vi "TDC_DAQV28_Paralled_muon.vi"(7 "address":string[](array[string])=["192.168.10.20"], 8 "error in (no error)":errorcluster, 9 "stop":bool, 10 "save data":bool=TRUE, 11 "SMA mode":bool) -> (0 "error out 3":errorcluster, 2 "csv path":path=path "G:/tdc/2017/data/test_20250303_062615.csv", 3 "rate":dbl=1.0935487223592613)   [LabVIEW 2017]
uses:
  gloabal.vi
  <vilib>/Utility/file.llb/Write Delimited Spreadsheet (DBL).vi
  <vilib>/Utility/file.llb/Write Delimited Spreadsheet (I64).vi
panel:
  out "cal 3":u32[](graph)=[0, 0, 0, 0, 0, 0, 0, 0, 0, 0, 0, 0, 0, 0, 0, 0, 0, 0, 0, 0, 0, 0, 0, 0, 0, 0, 0, 0, 0, 0, 0, 0, 0, 0, 0, 0, 0, 0, 0, 0, 0, 0, 0, 0, 0, 0, 0, 0, 0, 0, 0, 0, 0, 0, 0, 0, 0, 0, 0, 0, 0, 0, 0, 0, 0, 0, 0, 0, 0, 0, 0, 0, 0, 0, 0, 0, 0, 0, 0, 0, 0, 0, 0, 0, 0, 0, 0, 0, 0, 0, 0, 0, 0, 0, 0, 0, 0, 0, 0, 0, 0, 0, 0, 0, 0, 0, 0, 0, 0, 0, 0, 0, 0, 0, 0, 0, 0, 0, 0, 0, 0, 0, 0, 0, 0, 0, 0, 0, 0, 0, 0, 0, 0, 0, 0, 0, 0, 0, 0, 0, 0, 0, 0, 0, 0, 0, 0, 0, 0, 0, 0, 0, 0, 0, 0, 0, 0, 0, 0, 0, 0, 0, 0, 0, 0, 15, 3, 1, 14, 3, 31, 20, 16, 6, 1, 18, 12, 4, 29, 10, 8, 29, 2, 14, 4, 25, 7, 24, 4, 0, 1, 5, 8, 18, 22, 0, 4, 5, 0, 12, 9, 9, 20, 21, 4, 10, 13, 5, 21, 13, 14, 2, 6, 13, 1, 3, 5, 10, 20, 2, 3, 4, 3, 4, 2, 20, 13, 2, 5, 1, 3, 12, 4, 1, 14, 7, 5, 4, 1, 10, 2, 21, 14, 2, 5, 10, 4, 0, 11, 19, 6, 4, 1, 37, 1, 4, 2, 1, 10, 13, 4, 8, 10, 6, 9, 2, 0, 6, 8, 12, 3, 21, 5, 7, 8, 2, 3, 7, 17, 6, 5, 6, 4, 6, 0, 2, 1, 3, 10, 33, 7, 2, 6, 3, 7, 3, 2, 0, 12, 10, 11, 13, 13, 7, 3, 9, 6, 16, 0, 13, 5, 6, 3, 0, 5, 5, 7, 1, 10, 7, 13, 14, 5, 1, 12, 7, 1, 10, 2, 1, 14, 18, 13, 11, 4, 6, 9, 22, 11, 9, 2, 2, 8, 14, 4, 4, 6, 12, 13, 3, 9, 5, 5, 1, 5, 11, 18, 3, 0, 5, 4, 6, 7, 6, 1, 13, 5, 1, 2, 2, 1, 4, 12, 7, 3, 2, 3, 9, 11, 1, 20, 3, 4, 5, 5, 3, 5, 8, 5, 3, 26, 14, 6, 1, 3, 12, 12, 4, 23, 10, 3, 4, 4, 10, 3, 5, 4, 2, 14, 5, 15, 20, 1, 5, 1, 20, 6, 1, 3, 13, 21, 12, 7, 4, 1, 5, 30, 11, 2, 4, 0, 12, 7, 10, 3, 2, 25, 6, 1, 3, 6, 3, 8, 37, 4, 6, 2, 2, 4, 3, 5, 6, 13, 6, 9, 22, 1, 3, 7, 7, 4, 8, 33, 2, 1, 15, 3, 8, 23, 21, 2, 2, 27, 13, 3, 5, 10, 4, 18, 5, 5, 8, 0, 1, 8, 12, 4, 3, 0, 4, 8, 4, 7, 4, 2, 11, 13, 3, 0, 7, 5, 3, 4, 8, 4, 20, 2, 13, 4, 8, 6, 17, 4, 2, 1, 15, 2, 15, 5, 19, 0, 4, 15, 4, 16, 11, 1, 16, 4, 6, 6, 5, 7, 3, 9, 15, 3, 6, 3, 13, 5, 7, 3, 27, 2, 0, 21, 1, 4, 1, 4, 5, 3, 10, 7, 3, 6, 4, 18, 21, 7, 6, 7, 7, 12, 6, 9, 8, 11, 12, 13, 2, 2, 5, 4, 7, 52, 3, 5, 8, 7, 10, 4, 4, 6, 5, 18, 0, 3, 6, 1, 9, 5, 19, 13, 24, 12, 4, 4, 15, 6, 41, 3, 8, 5, 17, 26, 8, 7, 20, 2, 5, 12, 10, 10, 12, 9, 17, 6, 3, 1, 5, 3, 7, 8, 4, 10, 5, 10, 7, 1, 2, 14, 7, 25, 3, 0, 0, 0, 5, 21, 8, 14, 4, 10, 2, 3, 2, 4, 8, 12, 3, 6, 8, 3, 4, 3, 20, 5, 6, 7, 8, 11, 2, 8, 6, 5, 15, 17, 10, 10, 3, 3, 9, 18, 7, 7, 3, 5, 5, 5, 2, 2, 2, 4, 1, 0, 42, 3, 14, 4, 3, 5, 2, 7, 4, 2, 7, 5, 22, 4, 3, 17, 3, 5, 8, 19, 7, 5, 0, 3, 4, 10, 1, 8, 2, 2, 13, 23, 4, 9, 5, 0, 0, 0, 27, 2, 16, 11, 15, 3, 0, 18, 2, 8, 29, 19, 6, 7, 2, 6, 12, 1, 13, 2, 7, 5, 11, 8, 5, 6, 6, 19, 2, 4, 0, 7, 22, 13, 3, 7, 3, 8, 11, 0, 3, 26, 6, 5, 5, 6, 4, 10, 17, 16, 4, 3, 4, 3, 4, 21, 8, 10, 10, 7, 0, 9, 9, 2, 10, 10, 2, 9, 9, 4, 14, 5, 5, 4, 18, 6, 3, 0, 4, 1, 20, 2, 33, 4, 1, 2, 1, 20, 6, 3, 11, 10, 2, 1, 13, 9, 6, 1, 0, 0, 0, 0, 0, 0, 0, 0, 0, 0, 0, 0, 0, 0, 0, 0, 0, 0, 0, 0, 0, 0, 0, 0, 0, 0, 0, 0, 0, 0, 0, 0, 0, 0, 0, 0, 0, 0, 0, 0, 0, 0, 0, 0, 0, 0, 0, 0, 0, 0, 0, 0, 0, 0, 0, 0, 0, 0, 0, 0, 0, 0, 0, 0, 0, 0, 0, 0, 0, 0, 0, 0, 0, 0, 0, 0, 0, 0, 0, 0, 0, 0, 0, 0, 0, 0, 0, 0, 0, 0, 0, 0, 0, 0, 0, 0, 0, 0, 0, 0, 0, 0, 0, 0, 0, 0, 0, 0, 0, 0, 0, 0, 0, 0, 0, 0, 0, 0, 0, 0, 0, 0, 0, 0, 0, 0, 0, 0, 0, 0, 0, 0, 0, 0, 0, 0, 0, 0, 0, 0, 0, 0, 0, 0, 0, 0, 0, 0, 0, 0, 0, 0, 0, 0, 0, 0, 0, 0, 0, 0, 0, 0, 0, 0, 0, 0, 0, 0, 0, 0, 0, 0, 0, 0, 0, 0, 0, 0, 0, 0, 0, 0, 0, 0, 0, 0, 0, 0, 0, 0, 0, 0, 0, 0, 0, 0, 0, 0, 0, 0, 0, 0, 0, 0, 0, 0, 0, 0, 0, 0, 0, 0, 0, 0, 0, 0, 0, 0, 0, 0, 0, 0, 0, 0, 0, 0, 0, 0, 0, 0, 0, 0, 0, 0, 0, 0, 0, 0, 0, 0, 0, 0, 0, 0, 0, 0, 0, 0, 0, 0, 0, 0, 0, 0, 0, 0, 0, 0, 0, 0, 0, 0, 0, 0, 0, 0, 0, 0, 0, 0, 0, 0, 0, 0, 0, 0, 0, 0, 0, 0, 0, 0, 0, 0, 0, 0, 0, 0, 0, 0, 0, 0, 0, 0, 0, 0, 0, 0, 0, 0, 0, 0, 0, 0, 0, 0, 0, 0, 0, 0, 0, 0, 0, 0, 0, 0, 0, 0, 0, 0, 0, 0, 0, 0, 0, 0, 0, 0, 0, 0, 0, 0, 0, 0, 0, 0, 0, 0, 0, 0, 0, 0, 0, 0, 0, 0, 0, 0, 0, 0, 0, 0, 0, 0, 0, 0, 0, 0, 0, 0, 0, 0, 0, 0, 0, 0, 0, 0, 0, 0, 0, 0, 0, 0, 0, 0, 0, 0, 0, 0, 0, 0, 0, 0, 0, 0, 0, 0, 0, 0, 0, 0, 0, 0, 0, 0, 0, 0, 0, 0, 0, 0, 0, 0, 0, 0, 0, 0, 0, 0, 0, 0, 0, 0, 0, 0, 0, 0, 0, 0, 0, 0, 0, 0, 0, 0, 0, 0, 0, 0, 0, 0, 0, 0, 0, 0, 0, 0, 0, 0, 0, 0, 0, 0, 0, 0, 0, 0, 0, 0, 0, 0, 0, 0, 0, 0, 0, 0, 0, 0, 0, 0, 0, 0, 0, 0, 0, 0, 0, 0, 0, 0, 0, 0, 0, 0, 0, 0, 0, 0, 0, 0, 0, 0, 0, 0, 0, 0, 0, 0, 0, 0, 0, 0, 0, 0, 0, 0, 0, 0, 0, 0, 0, 0, 0, 0, 0, 0, 0, 0, 0, 0, 0, 0, 0, 0, 0, 0, 0, 0, 0, 0, 0, 0, 0, 0, 0, 0, 0, 0, 0, 0, 0, 0, 0, 0, 0, 0, 0, 0, 0, 0, 0, 0, 0, 0, 0, 0, 0, 0, 0, 0, 0, 0, 0, 0, 0, 0, 0, 0, 0, 0, 0, 0, 0, 0, 0, 0, 0, 0, 0, 0, 0, 0, 0, 0, 0, 0, 0, 0, 0, 0, 0, 0, 0, 0, 0, 0, 0, 0, 0, 0, 0, 0, 0, 0, 0, 0, 0, 0, 0, 0, 0, 0, 0, 0, 0, 0, 0, 0, 0, 0, 0, 0, 0, 0, 0, 0, 0, 0, 0, 0, 0, 0, 0, 0, 0, 0, 0, 0, 0, 0, 0, 0, 0, 0, 0, 0, 0, 0, 0, 0, 0, 0, 0, 0, 0, 0, 0, 0, 0, 0, 0, 0, 0, 0, 0, 0, 0, 0, 0, 0, 0, 0, 0, 0, 0, 0, 0, 0, 0, 0, 0, 0, 0, 0, 0, 0, 0, 0, 0, 0, 0, 0, 0, 0, 0, 0, 0, 0, 0, 0, 0, 0, 0, 0, 0, 0, 0, 0, 0, 0, 0, 0, 0, 0, 0, 0, 0, 0, 0, 0, 0, 0, 0, 0, 0, 0, 0, 0, 0, 0, 0, 0, 0, 0, 0, 0, 0, 0, 0, 0, 0, 0, 0, 0, 0, 0, 0, 0, 0, 0, 0, 0, 0, 0, 0, 0, 0, 0, 0, 0, 0, 0, 0, 0, 0, 0, 0, 0, 0, 0, 0, 0, 0, 0, 0, 0, 0, 0, 0, 0, 0, 0, 0, 0, 0, 0, 0, 0, 0, 0, 0, 0, 0, 0, 0, 0, 0, 0, 0, 0, 0, 0, 0, 0, 0, 0, 0, 0, 0, 0, 0, 0, 0, 0, 0, 0, 0, 0, 0, 0, 0, 0, 0, 0, 0, 0, 0, 0, 0, 0, 0, 0, 0, 0, 0, 0, 0, 0, 0, 0, 0, 0, 0, 0, 0, 0, 0, 0, 0, 0, 0, 0, 0, 0, 0, 0, 0, 0, 0, 0, 0, 0, 0, 0, 0, 0, 0, 0, 0, 0, 0, 0, 0, 0, 0, 0, 0, 0, 0, 0, 0, 0, 0, 0, 0, 0, 0, 0, 0, 0, 0, 0, 0, 0, 0, 0, 0, 0, 0, 0, 0, 0, 0, 0, 0, 0, 0, 0, 0, 0, 0, 0, 0, 0, 0, 0, 0, 0, 0, 0, 0, 0, 0, 0, 0, 0, 0, 0, 0, 0, 0, 0, 0, 0, 0, 0, 0, 0, 0, 0, 0, 0, 0, 0, 0, 0, 0, 0, 0, 0, 0, 0, 0, 0, 0, 0, 0, 0, 0, 0, 0, 0, 0, 0, 0, 0, 0, 0, 0, 0, 0, 0, 0, 0, 0, 0, 0, 0, 0, 0, 0, 0, 0, 0, 0, 0, 0, 0, 0, 0, 0, 0, 0, 0, 0, 0, 0, 0, 0, 0, 0, 0, 0, 0, 0, 0, 0, 0, 0, 0, 0, 0, 0, 0, 0, 0, 0, 0, 0, 0, 0, 0, 0, 0, 0, 0, 0, 0, 0, 0, 0, 0, 0, 0, 0, 0, 0, 0, 0, 0, 0, 0, 0, 0, 0, 0, 0, 0, 0, 0, 0, 0, 0, 0, 0, 0, 0, 0, 0, 0, 0, 0, 0, 0, 0, 0, 0, 0, 0, 0, 0, 0, 0, 0, 0, 0, 0, 0, 0, 0, 0, 0, 0, 0, 0, 0, 0, 0, 0, 0, 0, 0, 0, 0, 0, 0, 0, 0, 0, 0, 0, 0, 0, 0, 0, 0, 0, 0, 0, 0, 0, 0, 0, 0, 0, 0, 0, 0, 0, 0, 0, 0, 0, 0, 0, 0, 0, 0, 0, 0, 0, 0, 0, 0, 0, 0, 0, 0, 0, 0, 0, 0, 0, 0, 0, 0, 0, 0, 0, 0, 0, 0, 0, 0, 0, 0, 0, 0, 0, 0, 0, 0, 0, 0, 0, 0, 0, 0, 0, 0, 0, 0, 0, 0, 0, 0, 0, 0, 0, 0, 0, 0, 0, 0, 0, 0, 0, 0, 0, 0, 0, 0, 0, 0, 0, 0, 0, 0, 0, 0, 0, 0, 0, 0, 0, 0, 0, 0, 0, 0, 0, 0, 0, 0, 0, 0, 0, 0, 0, 0, 0, 0, 0, 0, 0, 0, 0, 0, 0, 0, 0, 0, 0]
  out "x+y":u64
  out "channel number 3":u64 format="%x"
  in  "coarse counter width":u16(ring) items=["29", "48"]
  out "name (unnamed)":string
  out "error out 5":errorcluster
  in  "timeout":dbl=300.0
  out "DAC":dbl=8094.0
  out "Out":u8=3 format="%.0x"
  out "fine 4":u64=356036515840 format="%x"
  out "fine 3":u64=1390767640 format="%x"
  out "channel number 2":u64 format="%x"
  out "substring 3":string
  out "fine 2":u64=347691910 format="%x"
  out "substring 2":string
  out "substring":string
  in  "gps":bool
  out "Year":string="2025"
  in  "factor":i32=128
  in  "displayCR":bool=TRUE
  in  "Counter Setting":dbl=100000.0 format="%#_13g"
  in  "replace dat":bool
  in  "append csv":bool=TRUE
  out "element":string
  out "fine":u64=749 format="%x"
  in  "UDP Config":bool=TRUE
  in  "data  path":path=path "G:/tdc/2017/data"
  out "cal 2":u64[](graph)
  in  "Thresholds (mV)":dbl[](array[numeric])=[580.0, 580.0, 580.0, 580.0, 600.0, 600.0, 600.0, 600.0, 580.0, 580.0, 600.0, 600.0, 600.0, 600.0, 600.0, 600.0, 580.0, 580.0, 600.0, 600.0, 600.0, 600.0, 600.0, 600.0, 580.0, 580.0, 600.0, 600.0, 600.0, 600.0, 600.0, 600.0, 600.0, 600.0, 600.0, 600.0, 600.0, 600.0, 600.0, 600.0, 600.0, 600.0, 600.0, 600.0, 600.0, 600.0, 600.0, 600.0, 600.0, 600.0, 600.0, 600.0, 600.0, 600.0, 600.0, 600.0, 600.0, 600.0, 600.0, 600.0, 600.0, 600.0, 600.0, 600.0]
  out "error out 2":errorcluster
  in  "display":bool=TRUE
  in  "Thresholds":dbl=-0.03
  in  "one key for threshold":bool=TRUE
  in  "RST":bool
  in  "通道数量":i32=128
  out "Cal Table":u32[](array[numeric])=[100002, 100002, 0, 0, 0, 0, 0, 0, 0, 0, 0, 0, 0, 0, 0, 0, 0, 0, 0, 0, 0, 0, 0, 0, 0, 0, 0, 0, 0, 0, 0, 0, 0, 0, 0, 0, 0, 0, 0, 0, 0, 0, 0, 0, 0, 0, 0, 0, 0, 0, 0, 0, 0, 0, 0, 0, 0, 0, 0, 0, 0, 0, 0, 0, 0, 0, 0, 0, 0, 0, 0, 0, 0, 0, 0, 0, 0, 0, 0, 0, 0, 0, 0, 0, 0, 0, 0, 0, 0, 0, 0, 0, 0, 0, 0, 0, 0, 0, 100002, 100002, 0, 0, 0, 0, 0, 0, 0, 0, 0, 0, 0, 0, 0, 0, 0, 0, 0, 0, 0, 0, 0, 0, 0, 0, 0, 0, 0, 0]
  in  "channel for cal":i32
  out "channel number":u64
  out "Calibration Counter":i32=100000
  out "Event index":i32=97959
  out "cal":u32[](graph)=[0, 0, 0, 0, 0, 0, 0, 0, 0, 0, 0, 0, 0, 0, 0, 0, 0, 0, 0, 0, 0, 0, 0, 0, 0, 0, 0, 0, 0, 0, 0, 0, 0, 0, 0, 0, 0, 0, 0, 0, 0, 0, 0, 0, 0, 0, 0, 0, 0, 0, 0, 0, 0, 0, 0, 0, 0, 0, 0, 0, 0, 0, 0, 0, 0, 0, 0, 0, 0, 0, 0, 0, 0, 0, 0, 0, 0, 0, 0, 0, 0, 0, 0, 0, 0, 0, 0, 0, 0, 0, 0, 0, 0, 0, 0, 0, 0, 0, 0, 0, 0, 0, 0, 0, 0, 0, 0, 0, 0, 0, 0, 0, 0, 0, 0, 0, 0, 0, 0, 0, 0, 0, 0, 0, 0, 0, 0, 0, 0, 0, 0, 0, 0, 0, 0, 0, 0, 0, 0, 0, 0, 0, 0, 0, 0, 0, 0, 0, 0, 0, 0, 0, 0, 0, 0, 0, 0, 0, 0, 0, 0, 0, 0, 0, 0, 15, 511, 47, 47, 496, 61, 99, 729, 29, 42, 171, 747, 96, 51, 42, 172, 695, 176, 314, 56, 529, 577, 49, 39, 32, 59, 217, 100, 54, 274, 367, 65, 147, 131, 182, 81, 199, 147, 352, 77, 542, 71, 254, 473, 91, 290, 270, 470, 39, 34, 220, 292, 32, 36, 306, 91, 30, 60, 270, 84, 115, 92, 342, 59, 193, 51, 55, 166, 178, 68, 201, 77, 48, 251, 157, 58, 175, 144, 73, 238, 174, 189, 202, 77, 49, 49, 85, 297, 134, 135, 191, 31, 343, 221, 39, 85, 162, 328, 62, 89, 210, 178, 65, 221, 260, 157, 46, 41, 35, 131, 307, 87, 392, 108, 46, 60, 293, 50, 28, 167, 101, 165, 43, 61, 148, 522, 39, 60, 263, 49, 52, 418, 91, 68, 40, 20, 504, 53, 95, 56, 124, 80, 60, 291, 176, 200, 307, 95, 332, 51, 42, 79, 81, 128, 130, 107, 114, 54, 243, 271, 151, 90, 157, 326, 162, 89, 139, 327, 44, 132, 379, 66, 138, 71, 729, 73, 135, 130, 269, 267, 206, 92, 141, 79, 58, 103, 46, 162, 368, 174, 84, 171, 248, 161, 88, 87, 85, 141, 71, 79, 100, 248, 53, 62, 46, 50, 29, 51, 151, 324, 134, 72, 55, 273, 116, 57, 432, 69, 101, 121, 112, 68, 129, 194, 50, 95, 235, 79, 432, 83, 320, 56, 85, 118, 185, 276, 83, 46, 247, 134, 161, 99, 82, 54, 346, 250, 66, 379, 111, 58, 47, 307, 58, 79, 133, 244, 54, 262, 133, 46, 43, 39, 274, 241, 171, 55, 222, 121, 72, 279, 53, 50, 69, 528, 61, 153, 48, 220, 139, 41, 384, 59, 142, 79, 150, 65, 43, 287, 51, 216, 69, 111, 314, 50, 328, 87, 107, 247, 222, 49, 113, 194, 307, 485, 52, 60, 292, 98, 760, 36, 82, 65, 80, 90, 182, 181, 48, 192, 40, 156, 51, 325, 87, 36, 31, 44, 140, 97, 82, 144, 162, 67, 335, 57, 34, 44, 107, 46, 49, 157, 326, 231, 52, 48, 325, 105, 61, 219, 47, 357, 66, 68, 245, 77, 106, 285, 61, 245, 39, 43, 236, 326, 164, 131, 73, 165, 77, 225, 56, 62, 45, 422, 137, 93, 81, 169, 47, 198, 173, 350, 60, 357, 57, 32, 55, 64, 54, 64, 147, 199, 199, 92, 169, 312, 172, 158, 231, 65, 129, 68, 243, 77, 214, 57, 316, 70, 86, 59, 128, 51, 39, 930, 119, 134, 78, 46, 106, 248, 87, 93, 90, 320, 90, 60, 76, 239, 138, 140, 375, 323, 460, 154, 50, 67, 245, 237, 687, 62, 74, 111, 420, 292, 99, 335, 396, 57, 225, 111, 125, 191, 131, 151, 340, 112, 74, 88, 108, 142, 215, 212, 62, 224, 110, 55, 62, 110, 67, 75, 331, 263, 111, 107, 156, 80, 35, 160, 178, 377, 128, 77, 200, 62, 55, 60, 185, 235, 153, 63, 102, 299, 52, 72, 427, 135, 66, 95, 93, 146, 410, 54, 135, 78, 207, 103, 114, 94, 379, 159, 137, 422, 82, 64, 49, 43, 48, 73, 426, 60, 46, 37, 39, 50, 329, 413, 120, 95, 108, 29, 66, 59, 254, 54, 62, 160, 117, 230, 100, 119, 290, 131, 164, 113, 145, 149, 109, 172, 90, 127, 129, 161, 60, 153, 140, 107, 110, 117, 131, 297, 70, 47, 399, 156, 187, 68, 61, 212, 125, 427, 52, 289, 198, 138, 147, 346, 170, 168, 330, 74, 71, 89, 314, 331, 132, 133, 97, 154, 80, 111, 135, 270, 207, 206, 349, 111, 57, 278, 56, 155, 199, 230, 49, 176, 311, 128, 140, 146, 205, 111, 202, 158, 309, 108, 180, 95, 107, 237, 174, 119, 149, 86, 87, 234, 78, 88, 101, 101, 247, 99, 131, 235, 140, 122, 39, 83, 64, 241, 51, 34, 52, 104, 13, 43, 35, 30, 7, 0, 0, 1, 0, 0, 0, 0, 0, 0, 0, 0, 0, 0, 0, 0, 0, 0, 0, 0, 0, 0, 0, 0, 0, 0, 0, 0, 0, 0, 0, 0, 0, 0, 0, 0, 0, 0, 0, 0, 0, 0, 0, 0, 0, 0, 0, 0, 0, 0, 0, 0, 0, 0, 0, 0, 0, 0, 0, 0, 0, 0, 0, 0, 0, 0, 0, 0, 0, 0, 0, 0, 0, 0, 0, 0, 0, 0, 0, 0, 0, 0, 0, 0, 0, 0, 0, 0, 0, 0, 0, 0, 0, 0, 0, 0, 0, 0, 0, 0, 0, 0, 0, 0, 0, 0, 0, 0, 0, 0, 0, 0, 0, 0, 0, 0, 0, 0, 0, 0, 0, 0, 0, 0, 0, 0, 0, 0, 0, 0, 0, 0, 0, 0, 0, 0, 0, 0, 0, 0, 0, 0, 0, 0, 0, 0, 0, 0, 0, 0, 0, 0, 0, 0, 0, 0, 0, 0, 0, 0, 0, 0, 0, 0, 0, 0, 0, 0, 0, 0, 0, 0, 0, 0, 0, 0, 0, 0, 0, 0, 0, 0, 0, 0, 0, 0, 0, 0, 0, 0, 0, 0, 0, 0, 0, 0, 0, 0, 0, 0, 0, 0, 0, 0, 0, 0, 0, 0, 0, 0, 0, 0, 0, 0, 0, 0, 0, 0, 0, 0, 0, 0, 0, 0, 0, 0, 0, 0, 0, 0, 0, 0, 0, 0, 0, 0, 0, 0, 0, 0, 0, 0, 0, 0, 0, 0, 0, 0, 0, 0, 0, 0, 0, 0, 0, 0, 0, 0, 0, 0, 0, 0, 0, 0, 0, 0, 0, 0, 0, 0, 0, 0, 0, 0, 0, 0, 0, 0, 0, 0, 0, 0, 0, 0, 0, 0, 0, 0, 0, 0, 0, 0, 0, 0, 0, 0, 0, 0, 0, 0, 0, 0, 0, 0, 0, 0, 0, 0, 0, 0, 0, 0, 0, 0, 0, 0, 0, 0, 0, 0, 0, 0, 0, 0, 0, 0, 0, 0, 0, 0, 0, 0, 0, 0, 0, 0, 0, 0, 0, 0, 0, 0, 0, 0, 0, 0, 0, 0, 0, 0, 0, 0, 0, 0, 0, 0, 0, 0, 0, 0, 0, 0, 0, 0, 0, 0, 0, 0, 0, 0, 0, 0, 0, 0, 0, 0, 0, 0, 0, 0, 0, 0, 0, 0, 0, 0, 0, 0, 0, 0, 0, 0, 0, 0, 0, 0, 0, 0, 0, 0, 0, 0, 0, 0, 0, 0, 0, 0, 0, 0, 0, 0, 0, 0, 0, 0, 0, 0, 0, 0, 0, 0, 0, 0, 0, 0, 0, 0, 0, 0, 0, 0, 0, 0, 0, 0, 0, 0, 0, 0, 0, 0, 0, 0, 0, 0, 0, 0, 0, 0, 0, 0, 0, 0, 0, 0, 0, 0, 0, 0, 0, 0, 0, 0, 0, 0, 0, 0, 0, 0, 0, 0, 0, 0, 0, 0, 0, 0, 0, 0, 0, 0, 0, 0, 0, 0, 0, 0, 0, 0, 0, 0, 0, 0, 0, 0, 0, 0, 0, 0, 0, 0, 0, 0, 0, 0, 0, 0, 0, 0, 0, 0, 0, 0, 0, 0, 0, 0, 0, 0, 0, 0, 0, 0, 0, 0, 0, 0, 0, 0, 0, 0, 0, 0, 0, 0, 0, 0, 0, 0, 0, 0, 0, 0, 0, 0, 0, 0, 0, 0, 0, 0, 0, 0, 0, 0, 0, 0, 0, 0, 0, 0, 0, 0, 0, 0, 0, 0, 0, 0, 0, 0, 0, 0, 0, 0, 0, 0, 0, 0, 0, 0, 0, 0, 0, 0, 0, 0, 0, 0, 0, 0, 0, 0, 0, 0, 0, 0, 0, 0, 0, 0, 0, 0, 0, 0, 0, 0, 0, 0, 0, 0, 0, 0, 0, 0, 0, 0, 0, 0, 0, 0, 0, 0, 0, 0, 0, 0, 0, 0, 0, 0, 0, 0, 0, 0, 0, 0, 0, 0, 0, 0, 0, 0, 0, 0, 0, 0, 0, 0, 0, 0, 0, 0, 0, 0, 0, 0, 0, 0, 0, 0, 0, 0, 0, 0, 0, 0, 0, 0, 0, 0, 0, 0, 0, 0, 0, 0, 0, 0, 0, 0, 0, 0, 0, 0, 0, 0, 0, 0, 0, 0, 0, 0, 0, 0, 0, 0, 0, 0, 0, 0, 0, 0, 0, 0, 0, 0, 0, 0, 0, 0, 0, 0, 0, 0, 0, 0, 0, 0, 0, 0, 0, 0, 0, 0, 0, 0, 0, 0, 0, 0, 0, 0, 0, 0, 0, 0, 0, 0, 0, 0, 0, 0, 0, 0, 0, 0, 0, 0, 0, 0, 0, 0, 0, 0, 0, 0, 0, 0, 0, 0, 0, 0, 0, 0, 0, 0, 0, 0, 0, 0, 0, 0, 0, 0, 0, 0, 0, 0, 0, 0, 0, 0, 0, 0, 0, 0, 0, 0, 0, 0, 0, 0, 0, 0, 0, 0, 0, 0, 0, 0, 0, 0, 0, 0, 0, 0, 0, 0, 0, 0, 0, 0, 0, 0, 0, 0, 0, 0, 0, 0, 0, 0, 0, 0, 0, 0, 0, 0, 0, 0, 0, 0, 0, 0, 0, 0, 0, 0, 0, 0, 0, 0, 0, 0, 0, 0, 0, 0, 0, 0, 0, 0, 0, 0, 0, 0, 0, 0, 0, 0, 0, 0, 0, 0, 0, 0, 0, 0, 0, 0, 0, 0, 0, 0, 0, 0, 0, 0, 0, 0, 0, 0, 0, 0, 0, 0, 0, 0, 0, 0, 0, 0, 0, 0, 0, 0, 0, 0, 0, 0, 0, 0, 0, 0, 0, 0, 0, 0, 0, 0, 0, 0, 0, 0, 0, 0, 0, 0, 0, 0, 0, 0, 0, 0, 0, 0, 0, 0, 0, 0, 0, 0, 0, 0, 0, 0, 0, 0, 0, 0, 0, 0, 0, 0, 0, 0, 0, 0, 0, 0, 0, 0, 0, 0, 0, 0, 0, 0, 0, 0, 0, 0, 0, 0, 0, 0, 0, 0, 0, 0, 0, 0, 0, 0, 0, 0, 0, 0, 0, 0, 0, 0, 0, 0, 0, 0, 0, 0, 0, 0, 0, 0, 0, 0, 0, 0, 0, 0, 0, 0, 0, 0, 0, 0, 0, 0, 0, 0, 0, 0, 0, 0, 0, 0, 0, 0, 0, 0, 0, 0, 0, 0, 0, 0, 0, 0, 0, 0, 0, 0, 0, 0, 0, 0, 0, 0, 0, 0, 0, 0, 0, 0, 0, 0, 0, 0, 0, 0, 0, 0, 0, 0, 0, 0, 0, 0, 0, 0, 0, 0, 0, 0, 0, 0, 0, 0, 0, 0, 0, 0, 0, 0, 0, 0, 0, 0, 0, 0, 0, 0, 0, 0, 0, 0, 0, 0, 0, 0, 0, 0, 0, 0, 0, 0, 0, 0, 0, 0, 0, 0, 0, 0, 0, 0, 0, 0, 0, 0, 0, 0, 0, 0, 0, 0, 0, 0, 0, 0, 0, 0, 0, 0, 0, 0, 0, 0, 0, 0, 0, 0, 0, 0, 0, 0, 0, 0, 0, 0, 0, 0, 0, 0, 0, 0, 0, 0, 0, 0, 0, 0, 0, 0, 0, 0, 0, 0, 0, 0, 0, 0, 0, 0, 0, 0, 0, 0, 0, 0, 0, 0, 0, 0, 0, 0, 0, 0, 0, 0, 0, 0, 0, 0, 0, 0, 0, 0, 0, 0, 0, 0, 0, 0, 0, 0, 0, 0, 0, 0, 0, 0, 0, 0, 0, 0, 0, 0, 0, 0, 0, 0, 0, 0, 0, 0, 0, 0, 0, 0, 0, 0, 0, 0, 0, 0, 0, 0, 0, 0, 0, 0, 0, 0, 0, 0, 0, 0, 0]
  out "error out":errorcluster
  out "appended path":path=path "G:/tdc/2017/data/test_20250303_062615.dat"
  in  "filename":string="test"
  in  "Events":i32=110000 min=1
  in  "timeout (ms)":i32=10000
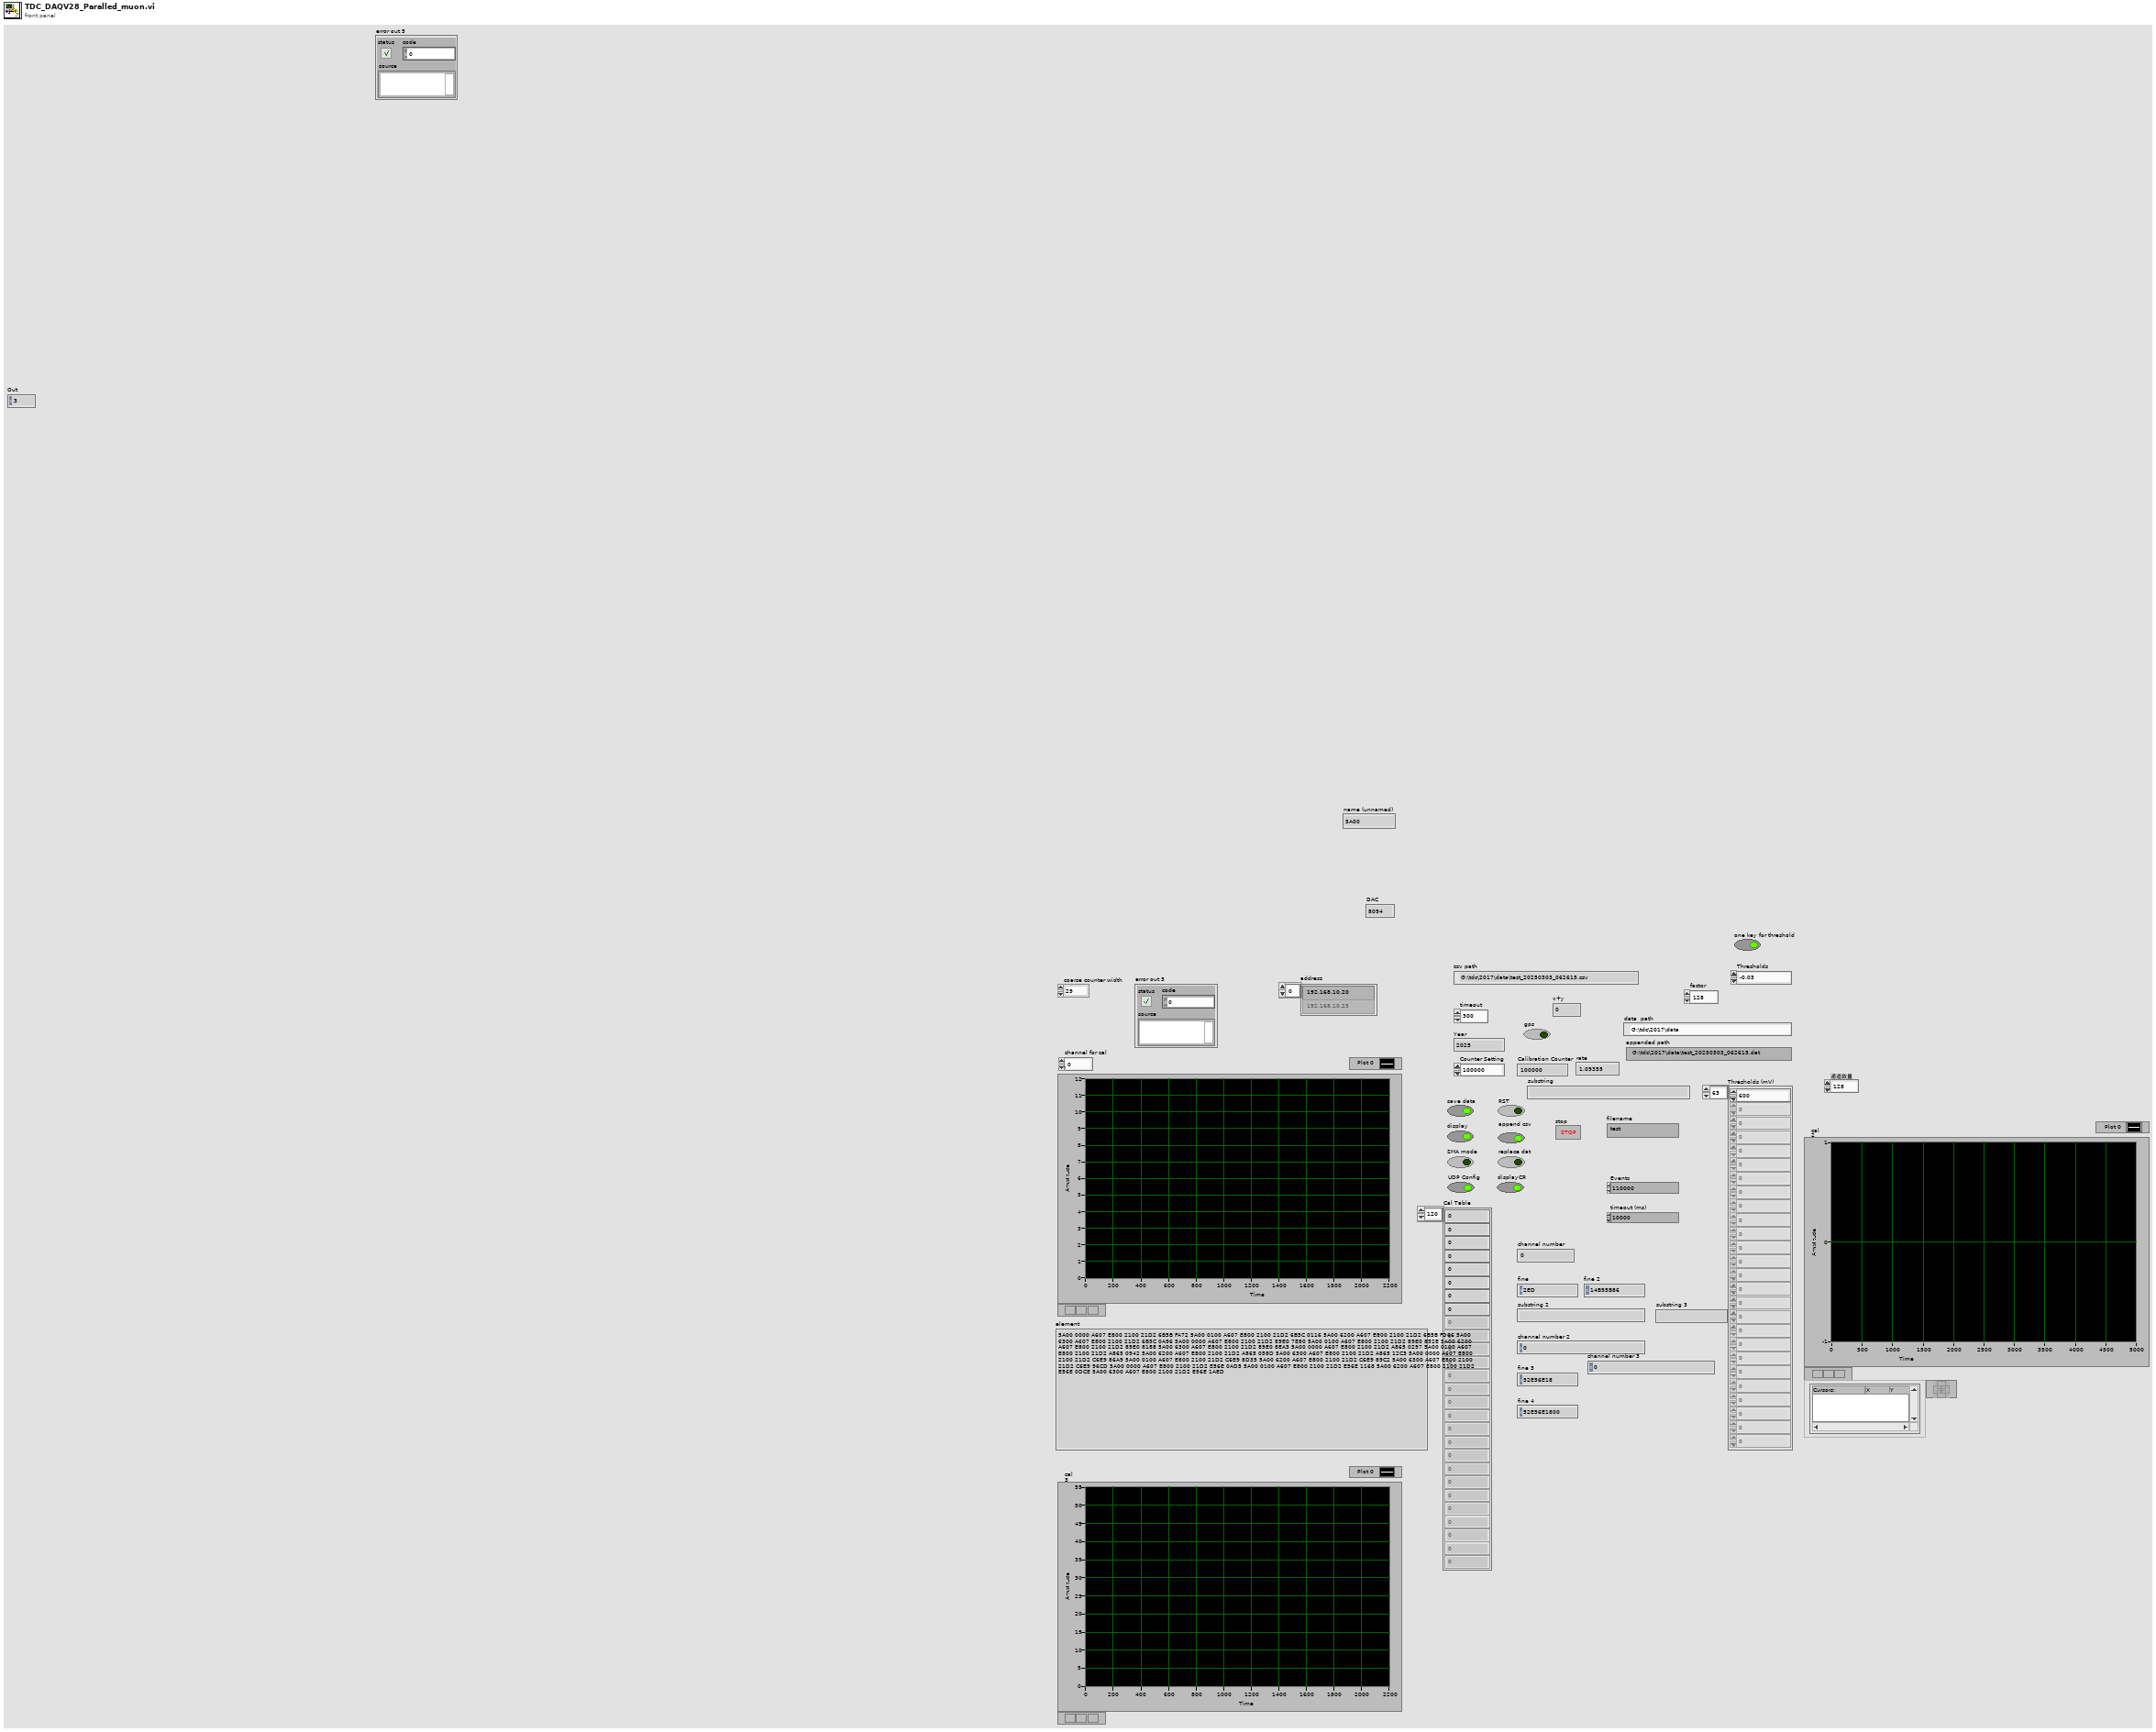
[diagram p1: front panel]
types:
  T1 = enum16{"open", "replace", "create", "open or create", "replace or create", "replace or create with confirmation"}
  T2 = enum16{"big-endian, network order", "native, host order", "little-endian"}
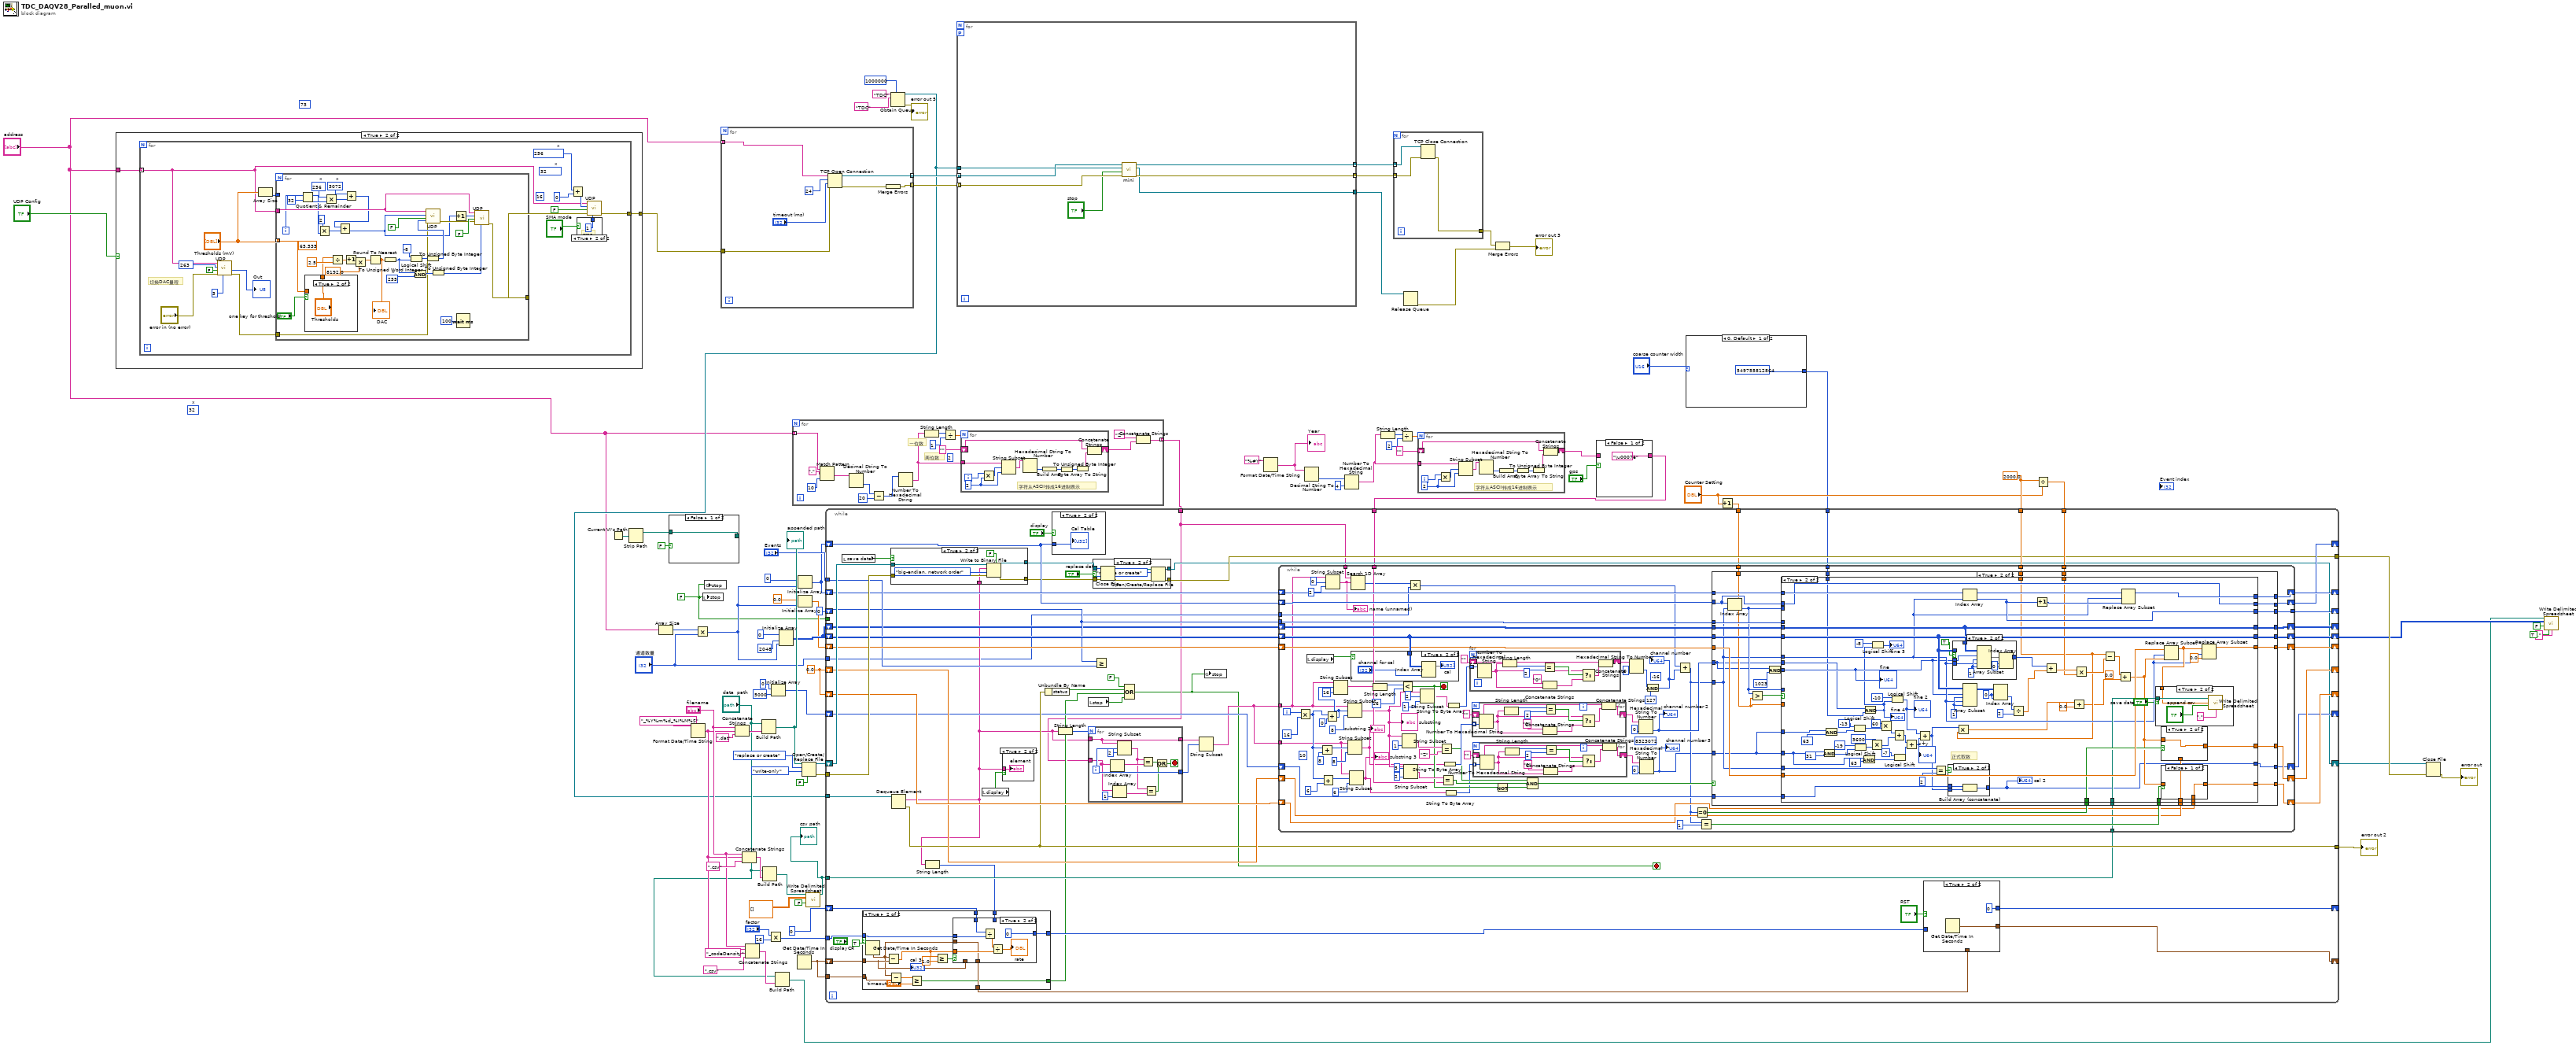
[diagram p0: block diagram]
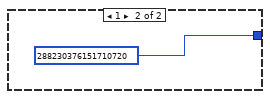
[diagram p2: hidden frame]
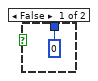
[diagram p5: hidden frame]
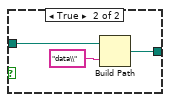
[diagram p7: hidden frame]
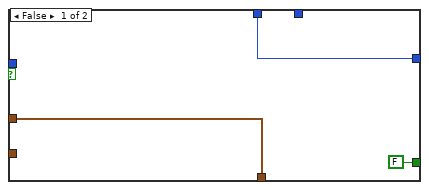
[diagram p11: hidden frame]
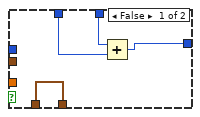
[diagram p12: hidden frame]
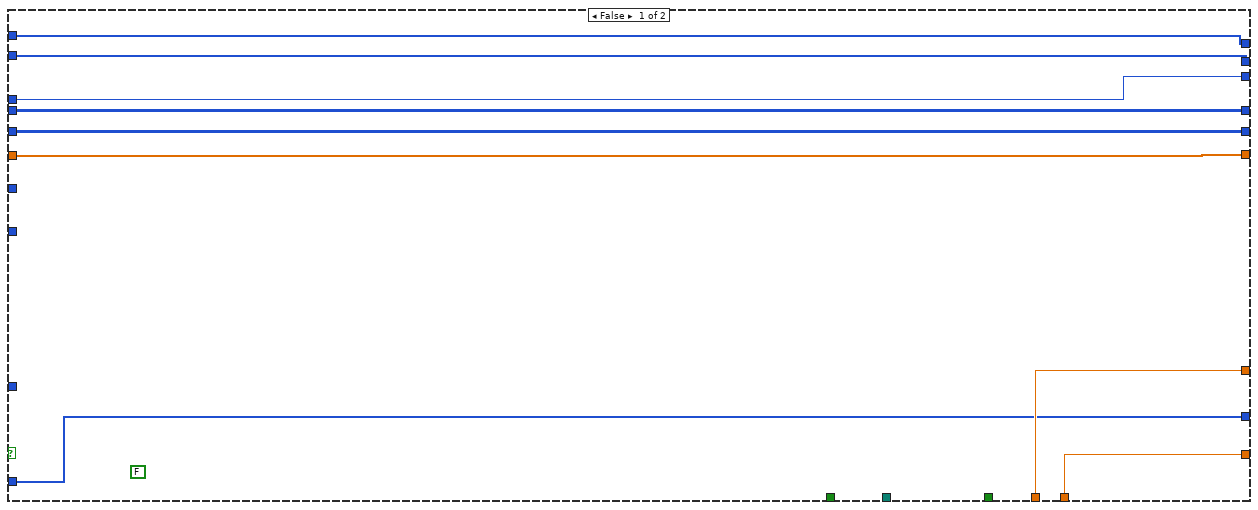
[diagram p16: hidden frame]
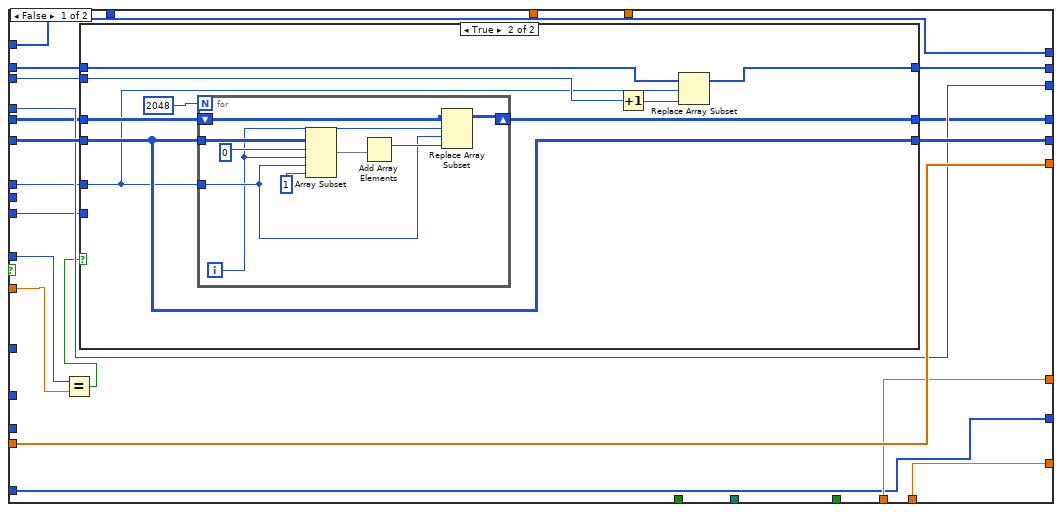
[diagram p17: hidden frame]
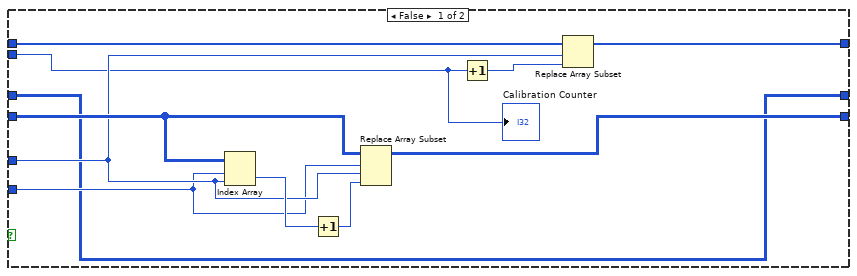
[diagram p18: hidden frame]
diagram:
  (unwired) u32 73 ("Address")
  w45 = 2000.0 ("x")
  (unwired) u16 32  # x
  w4 = FALSE ("stop")
  w69 = 0.0
  n1 = case shown="True" "UDP Config" {
    tunnel: "address" -> [_ w91]
    tunnel: [_ w92] -> w12
    frame False {
    }
    frame True {
      n2 = for {
        tunnel: [w107] -> w92
        tunnel: w91 -> [w95] mode=indexing
        (unwired) u16 32  # x
        (unwired) u32 16 ("Address")
        w100 = u16 256  # x
        # "切换DAC量程"
        n3 = call "UDP.vi"("In"=u8 3, "error in (no error)"="error in (no error)", "Read (TRUE)"=FALSE, "Address"=u32 263, "IP address"=w95) -> ("error out"=w93:errorcluster, "Out"=→"Out":u8)  [unwired: 4 in]
        n4 = Array Size(array="Thresholds (mV)") -> (size(s)=w104:i32)
        n5 = for {
          tunnel: w95 -> [w141]
          tunnel: "Thresholds (mV)" -> [w128] mode=indexing
          tunnel: [w131] -> w108
          tunnel: w104 -> [_]
          tunnel: w93 -> [w115]
          i -> [w123]
          (unwired) 65.535 ("y")
          w124 = u16 3072  # x
          w125 = u16 256  # x
          w137 = u16 255  # x
          n6 = Quotient & Remainder(x=w123, y=32) -> (x-y*floor(x/y)=w117:i32, floor(x/y)=w126:i32)
          n7 = case shown="True" "one key for threshold" {
            tunnel: [w147 "Thresholds"] -> w129
            tunnel: w128 -> [w147 _]
            frame False {
            }
            frame True {
            }
          }
          n8 = Multiply(x=2, y=w117) -> (x*y=w118:i32)
          n9 = Multiply(x=w125, y=w126) -> (x*y=w120:i32)
          n10 = Divide(x=w129, y=2.5) -> (x/y=w144:dbl)
          n11 = Increment(x=w144) -> (x+1=w114:dbl)
          n12 = Add(x=w124, y=w120) -> (x+y=w119:i32)
          n13 = Add(x=w119, y=w118) -> (x+y=w122:i32)
          n14 = Multiply(x=w114, y=8192.0) -> (x*y=w113:dbl)
          n15 = Round To Nearest(number=w113) -> (nearest integer value=w142:dbl)
          "DAC" <- w142
          n16 = To Unsigned Word Integer(number=w142) -> (unsigned 16bit integer=w133:u16)
          n17 = Logical Shift(y=i16 -8, x=w133) -> (x << y=w139:u16)
          n18 = And(x=w133, y=w137) -> (x .and. y?=w136:u16)
          n19 = To Unsigned Byte Integer(number=w139) -> (unsigned 8bit integer=w138:u8)
          n20 = call "UDP.vi"("In"=w138, "error in (no error)"=w115, "Read (TRUE)"=FALSE, "Address"=w122, "IP address"=w141) -> ("error out"=w132:errorcluster)  [unwired: 4 in, 1 out]
          n21 = To Unsigned Byte Integer(number=w136) -> (unsigned 8bit integer=w135:u8)
          n22 = Increment(x=w122) -> (x+1=w121:i32)
          n23 = Wait (ms)(milliseconds to wait=u32 100) -> ()  [unwired: 1 out]
          n24 = call "UDP.vi"("In"=w135, "error in (no error)"=w132, "Read (TRUE)"=FALSE, "Address"=w121, "IP address"=w141) -> ("error out"=w131:errorcluster)  [unwired: 4 in, 1 out]
        }
        n25 = Add(x=w100, y=u32 0 ("Address")) -> (x+y=w101:u32)
        n26 = case shown="True" "SMA mode" {
          tunnel: [u8 0 ("In") u8 1 ("In")] -> w106
          frame False {
          }
          frame True {
            # "sma"
          }
        }
        n27 = call "UDP.vi"("In"=w106, "error in (no error)"=w108, "Read (TRUE)"=FALSE, "Address"=w101, "IP address"=w95) -> ("error out"=w107:errorcluster)  [unwired: 4 in, 1 out]
      }
    }
  }
  n28 = Current VI's Path() -> (path=w85:path)
  n29 = Strip Path(path=w85) -> (stripped path=w84:path)  [unwired: 1 out]
  n30 = Array Size(array="address") -> (size(s)=w7:i32)
  n31 = case shown="False" FALSE {
    tunnel: w84 -> [w149 w151]
    tunnel: [w149 w150] -> _
    frame False {
    }
    frame True {
      n32 = Build Path(base path=w151, name or relative path="data\\") -> (appended path=w150:path)
    }
  }
  n33 = Format Date/Time String(time format string (%c)="_%Y%m%d_%I%M%S") -> (date/time string=w62:string)  [unwired: 2 in]
  n34 = Multiply(x=w7, y="通道数量") -> (x*y=w6:i32)
  n35 = local write "stop"(w4) -> ()
  n36 = global write "gloabal.vi" "stop"(w4) -> ()
  n37 = for {
    tunnel: "address" -> [w158] mode=indexing
    tunnel: [w157] -> w22 mode=indexing
    tunnel: [w155] -> w21 mode=indexing
    tunnel: w12 -> [w154]
    n38 = TCP Open Connection(address=w158, remote port or service name=u16 24 ("port"), timeout ms (60000)="timeout (ms)", error in (no error)=w154) -> (connection ID=w157:refnum<k5>, error out=w156:errorcluster)  [unwired: 1 in]
    n39 = Merge Errors(w156) -> (w155:errorcluster)
  }
  n40 = Concatenate Strings("filename", w62, ".dat") -> (w83:string)
  n41 = Concatenate Strings("filename", w62, ".csv") -> (w71:string)
  n42 = Concatenate Strings("filename", w62, "_codeDensity" ("string"), ".csv") -> (w59:string)
  n43 = Build Path(base path="data  path", name or relative path=w83) -> (appended path=w82:path)
  "appended path" <- w82
  n44 = Build Path(base path="data  path", name or relative path=w71) -> (appended path=w66:path)
  n45 = Multiply(x="factor", y=16) -> (x*y=w38:i32)
  n46 = Initialize Array(u32 0 ("element"), 5000 ("dimension size")) -> (w50:u32[])
  n47 = Build Path(base path="data  path", name or relative path=w59) -> (appended path=w56:path)
  n48 = Initialize Array(u32 0 ("element"), 2048 ("dimension size"), w6) -> (w68:u32[][])
  n49 = for {
    tunnel: [w161] -> w24 mode=indexing
    tunnel: "address" -> [w160] mode=indexing
    (unwired) 2 ("y")
    # "一位数"
    # "两位数"
    n50 = Match Pattern(string=w160, regular expression="." ("search string"), offset (0)=10) -> (after substring=w167:string)  [unwired: 3 out]
    n51 = Decimal String To Number(string=w167) -> (number=w164:i32)  [unwired: 2 in, 1 out]
    n52 = Subtract(x=w164, y=20) -> (x-y=w163:i32)
    n53 = Number To Hexadecimal String(2:w163) -> (0:w166:string)  [unwired: 1 in]
    n54 = String Length(string=w166) -> (length=w172:i32)
    n55 = Divide(x=w172, y=1) -> (x/y=w173:dbl)
    n56 = for {
      N: w173 -> [_]
      shift-right: [w185] -> w162
      shift-left: "" ("format string") -> [w184]
      tunnel: w166 -> [w175]
      i -> [w183]
      w177 = 2 ("y")
      # "字符从ASCII转成16进制表示"
      n57 = Multiply(x=w183, y=w177) -> (x*y=w176:i32)
      n58 = String Subset(string=w175, offset (0)=w176, length (rest)=w177) -> (substring=w178:string)
      n59 = Hexadecimal String To Number(string=w178) -> (number=w182:u32)  [unwired: 2 in, 1 out]
      n60 = Build Array(w182) -> (w181:u32[])
      n61 = To Unsigned Byte Integer(number=w181) -> (unsigned 8bit integer=w180:u8[])
      n62 = Byte Array To String(unsigned byte array=w180) -> (string=w179:string)
      n63 = Concatenate Strings(w184, w179) -> (w185:string)
    }
    n64 = Concatenate Strings("Z", w162) -> (w161:string)
  }
  n65 = Get Date/Time In Seconds() -> (seconds since 1Jan1904=w23:timestamp)
  n66 = Initialize Array(u32 0 ("element"), w6) -> (w70:u32[])
  n67 = Initialize Array(0.0, w6) -> (w52:dbl[])
  n68 = Open/Create/Replace File(file path (use dialog)=w82, operation (0:open)=T1."replace or create", access (0:read/write)=enum16{"read/write", "read-only", "write-only"}."write-only", disable buffering (F)=FALSE) -> (refnum out=w87:refnum<file>, error out=w86:errorcluster)  [unwired: 2 in, 1 out]
  n69 = call-poly <vilib>:"Write Delimited Spreadsheet.vi"("file path (dialog if empty)"=w66, "2D data"=dbl[][] [], "append to file? (new file:F)"=FALSE) -> ("new file path (Not A Path if cancelled)"=w3:path)  [unwired: 11 in, 1 out]
  "csv path" <- w3
  n70 = Obtain Queue(max queue size (-1, unlimited)=1000000, name (unnamed)="TDC", element data type="TDC" ("name (unnamed)")) -> (queue out=w13:refnum<queue>, error out=→"error out 5":errorcluster)  [unwired: 2 in, 1 out]
  n71 = for {
    tunnel: w22 -> [w192] mode=indexing
    tunnel: w21 -> [w191] mode=indexing
    tunnel: [w190] -> w20 mode=indexing
    tunnel: [w189] -> w19 mode=indexing
    workers-P: _ -> [_]
    tunnel: w13 -> [w188]
    tunnel: [w187] -> w14
    n72 = call "mini.vi"("error in (no error)"=w191, "stop"="stop", "queue out 2"=w188, "connection ID 2"=w192) -> ("error out 3"=w189:errorcluster, "queue out"=w187:refnum<queue>, "connection ID"=w190:refnum<k5>)  [unwired: 5 in]
  }
  n73 = Format Date/Time String(time format string (%c)="%#Y") -> (date/time string=w35:string)  [unwired: 2 in]
  "Year" <- w35
  n74 = Decimal String To Number(string=w35) -> (number=w34:i32)  [unwired: 2 in, 1 out]
  n75 = Number To Hexadecimal String(1:i16 4 ("width (-)"), 2:w34) -> (0:w28:string)
  n76 = String Length(string=w28) -> (length=w30:i32)
  n77 = for {
    tunnel: w20 -> [w195] mode=indexing
    tunnel: w19 -> [w194] mode=indexing
    tunnel: [w193] -> w11
    n78 = TCP Close Connection(connection ID=w195, error in (no error)=w194) -> (error out=w193:errorcluster)  [unwired: 1 in, 1 out]
  }
  n79 = Divide(x=w30, y=2) -> (x/y=w31:dbl)
  n80 = Release Queue(queue=w14) -> (error out=w10:errorcluster)  [unwired: 2 in, 2 out]
  n81 = for {
    N: w31 -> [_]
    shift-right: [w206] -> w27
    shift-left: "" ("format string") -> [w205]
    tunnel: w28 -> [w196]
    i -> [w204]
    w198 = 2 ("y")
    # "字符从ASCII转成16进制表示"
    n82 = Multiply(x=w204, y=w198) -> (x*y=w197:i32)
    n83 = String Subset(string=w196, offset (0)=w197, length (rest)=w198) -> (substring=w199:string)
    n84 = Hexadecimal String To Number(string=w199) -> (number=w203:u32)  [unwired: 2 in, 1 out]
    n85 = Build Array(w203) -> (w202:u32[])
    n86 = To Unsigned Byte Integer(number=w202) -> (unsigned 8bit integer=w201:u8[])
    n87 = Byte Array To String(unsigned byte array=w201) -> (string=w200:string)
    n88 = Concatenate Strings(w205, w200) -> (w206:string)
  }
  n89 = Merge Errors(w11, w10) -> (→"error out 3":errorcluster)
  n90 = case shown="False" "gps" {
    tunnel: w27 -> [_ w208]
    tunnel: ["\u0007è" ("format string") w208] -> w26
    frame False {
    }
    frame True {
    }
  }
  n91 = case shown="0, Default" "coarse counter width" {
    tunnel: [u64 549755812864 ("port") u64 288230376151710720 ("port")] -> w1
    frame 0, Default {
    }
    frame 1 {
    }
  }
  n92 = Increment(x="Counter Setting") -> (x+1=w41:dbl)
  n93 = Divide(x=w45, y="Counter Setting") -> (x/y=w44:dbl)
  n94 = while {
    tunnel: w86 -> [w270]
    tunnel: [w245] -> w53
    tunnel: [w234] -> w79
    shift-right: [w267] -> w57
    shift-left: w68 -> [w268]
    shift-right: [w254] -> _
    shift-left: w52 -> [w266]
    tunnel: "Events" -> [w265]
    shift-right: [w264] -> _
    shift-left: w70 -> [w263]
    shift-right: [w262] -> _
    shift-left: u32 0 ("element") -> [w261]
    shift-right: [w260] -> _
    shift-left: w70 -> [w247]
    shift-right: [w259] -> _
    shift-left: w69 -> [w256]
    shift-right: [w258] -> _
    shift-left: w69 -> [w257]
    shift-right: [w249] -> _
    shift-left: w68 -> [w255]
    tunnel: w3 -> [w241]
    shift-right: [w253] -> _
    shift-left: 0 -> [w228]
    shift-right: [w251] -> _
    shift-left: w23 -> [w250]
    tunnel: w4 -> [_]
    tunnel: w13 -> [w246]
    shift-right: [w242] -> _
    shift-left: w50 -> [w243]
    tunnel: w24 -> [w214]
    tunnel: w45 -> [w239]
    tunnel: w44 -> [w238]
    shift-right: [w233] -> w43
    shift-left: w87 -> [w269]
    tunnel: w41 -> [w232]
    tunnel: w38 -> [w225]
    tunnel: w26 -> [w222]
    tunnel: w23 -> [w221]
    tunnel: "通道数量" -> [w215]
    tunnel: w1 -> [w211]
    stop <- w213 stop-if-true
    n95 = local read "save data"() -> (w227:bool)
    n96 = Dequeue Element(queue=w246) -> (element=w217:string, error out=w245:errorcluster)  [unwired: 2 in, 2 out]
    n97 = case shown="True" w227 {
      tunnel: w270 -> [w283 w291]
      tunnel: w269 -> [w284 w290]
      tunnel: w217 -> [_ w287]
      tunnel: [w284 w286] -> w237
      tunnel: [w283 w285] -> w235
      frame False {
      }
      frame True {
        n98 = Write to Binary File(file (use dialog)=w290, data=w287, error in=w291, 5:FALSE ("prepend array or string size? (T)"), 9:T2."big-endian, network order" ("byte order (0:big-endian, network order)")) -> (refnum out=w286:refnum<file>, error out=w285:errorcluster)  [unwired: 1 in, 1 out]
      }
    }
    n99 = String Length(string=w217) -> (length=w229:i32)
    n100 = case shown="True" TRUE {
      tunnel: w250 -> [w303 w313]
      tunnel: [w303 w314] -> w231
      tunnel: w228 -> [w302 w312]
      tunnel: w229 -> [_ w311]
      tunnel: [w302 w310] -> w230
      tunnel: w225 -> [_ w309]
      tunnel: w221 -> [_ w307]
      tunnel: [FALSE w304] -> w220
      frame False {
      }
      frame True {
        n101 = Get Date/Time In Seconds() -> (seconds since 1Jan1904=w308:timestamp)
        n102 = Subtract(x=w308, y=w313) -> (x-y=w316:dbl)
        n103 = Subtract(x=w308, y=w307) -> (x-y=w306:dbl)
        n104 = Greater Or Equal?(x=w306, y="timeout") -> (x >= y?=w304:bool)
        n105 = Greater Or Equal?(x=w316, y=1.0) -> (x >= y?=w317:bool)
        n106 = case shown="True" w317 {
          tunnel: w316 -> [_ w328]
          tunnel: w308 -> [_ w326]
          tunnel: [w321 w326] -> w314
          tunnel: w313 -> [w321 _]
          tunnel: w312 -> [w320 w323]
          tunnel: w311 -> [w319 _]
          tunnel: [w318 0] -> w310
          tunnel: w309 -> [_ w322]
          frame False {
            n107 = Add(x=w319, y=w320) -> (x+y=w318:i32)
          }
          frame True {
            n108 = Divide(x=w323, y=w322) -> (x/y=w325:dbl)
            n109 = Divide(x=w325, y=w328) -> (x/y=→"rate":dbl)
          }
        }
      }
    }
    n110 = local read "display"() -> (w226:bool)
    n111 = case shown="True" w226 {
      tunnel: w217 -> [_ w282]
      frame False {
      }
      frame True {
        "element" <- w282
      }
    }
    n112 = Unbundle By Name(w245) -> ("status"=w244:bool)
    n113 = case shown="True" "display" {
      tunnel: w247 -> [_ w329]
      frame False {
      }
      frame True {
        "Cal Table" <- w329
      }
    }
    n114 = String Length(string=w217) -> (length=w219:i32)
    n115 = local read "stop"() -> (w212:bool)
    n116 = for {
      N: w219 -> [_]
      tunnel: w217 -> [w279]
      tunnel: [w279] -> w218
      tunnel: [w278] -> w216
      tunnel: w214 -> [w276]
      i -> [w278]
      stop <- w272 stop-if-true
      n117 = Index Array(array=w276) -> (element=w277:string)  [unwired: 1 in]
      n118 = Index Array(array=w276, index=1) -> (element=w274:string)
      n119 = String Subset(string=w279, offset (0)=w278, length (rest)=2 ("length (rest)")) -> (substring=w273:string)
      n120 = Equal?(x=w273, y=w277) -> (x = y?=w280:bool)
      n121 = Equal?(x=w273, y=w274) -> (x = y?=w271:bool)
      n122 = Or(x=w280, y=w271) -> (x .or. y?=w272:bool)
    }
    n123 = case shown="True" "replace dat" {
      tunnel: w237 -> [w293 w299]
      tunnel: [w293 w298] -> w233
      tunnel: w235 -> [w292 w295]
      tunnel: [w292 w294] -> w234
      frame False {
      }
      frame True {
        n124 = Close File(refnum=w299, error in=w295) -> (path=w300:path, error out=w296:errorcluster)
        n125 = Open/Create/Replace File(file path (use dialog)=w300, error in=w296, operation (0:open)=T1."replace or create") -> (refnum out=w298:refnum<file>, error out=w294:errorcluster)  [unwired: 3 in, 1 out]
      }
    }
    n126 = Greater Or Equal?(x=w261, y=w265) -> ()  [unwired: 1 out]
    n127 = Compound Arithmetic op=OR(FALSE ("x"), w244, w220, w212) -> (w213:bool)
    n128 = String Subset(string=w218, offset (0)=w216) -> (substring=w223:string)  [unwired: 1 in]
    n129 = global write "gloabal.vi" "stop"(w213) -> ()
    n130 = while {
      tunnel: w223 -> [w339]
      shift-right: [w417] -> w267
      shift-left: w268 -> [w415]
      shift-right: [w413] -> w254
      shift-left: w266 -> [w414]
      shift-right: [w410] -> w264
      shift-left: w263 -> [w409]
      tunnel: [w408] -> w262
      tunnel: w261 -> [w407]
      shift-right: [w405] -> w260
      shift-left: w247 -> [w406]
      shift-right: [w401] -> w259
      shift-left: w256 -> [w399]
      shift-right: [w397] -> w258
      shift-left: w257 -> [w398]
      tunnel: w241 -> [w396]
      shift-right: [w395] -> w249
      shift-left: w255 -> [w365]
      shift-right: [w392] -> w242
      shift-left: w243 -> [w393]
      tunnel: w223 -> [w358]
      tunnel: w239 -> [w372]
      tunnel: w238 -> [w371]
      tunnel: w232 -> [w364]
      tunnel: w222 -> [w353]
      tunnel: w215 -> [w341]
      tunnel: w214 -> [w340]
      tunnel: w211 -> [w335]
      i -> [w418]
      stop <- w367 stop-if-true
      (unwired) 10 ("length (rest)")
      (unwired) u64 8323072 ("port")
      (unwired) i16 -16 ("y")
      n131 = Multiply(x=w418, y=16 ("length (rest)")) -> (x*y=w359:i32)
      n132 = local read "display"() -> (w394:bool)
      n133 = Add(x=w359, y=8 ("length (rest)")) -> (x+y=w384:i32)
      n134 = Add(x=w359, y=6 ("length (rest)")) -> (x+y=w361:i32)
      n135 = Add(x=w359, y=0 ("length (rest)")) -> (x+y=w370:i32)
      n136 = String Subset(string=w339, offset (0)=0, length (rest)=2 ("length (rest)")) -> (substring=w342:string)
      "name (unnamed)" <- w342
      n137 = String Subset(string=w339, offset (0)=w370, length (rest)=16 ("y")) -> (substring=w368:string)
      n138 = String Subset(string=w339, offset (0)=w370, length (rest)=8 ("length (rest)")) -> (substring=w351:string)
      "substring" <- w351
      n139 = String Subset(string=w358, offset (0)=w384, length (rest)=8 ("length (rest)")) -> (substring=w348:string)
      "substring 2" <- w348
      n140 = String Subset(string=w358, offset (0)=w361, length (rest)=6 ("length (rest)")) -> (substring=w347:string)
      "substring 3" <- w347
      n141 = Search 1D Array(1D array=w340, element=w342) -> (index of element=w343:i32)  [unwired: 1 in]
      n142 = case shown="True" w394 {
        tunnel: w415 -> [_ w444]
        frame False {
        }
        frame True {
          n143 = Index Array(array=w444, index (col)="channel for cal") -> (element=→"cal":u32[])  [unwired: 1 in]
        }
      }
      n144 = String Length(string=w368) -> (length=w412:i32)
      n145 = Less?(x=w412, y=16) -> (x < y?=w367:bool)
      n146 = String Subset(string=w351, length (rest)=1 ("length (rest)")) -> (substring=w389:string)  [unwired: 1 in]
      n147 = String Subset(string=w351, offset (0)=5, length (rest)=2 ("length (rest)")) -> (substring=w373:string)
      n148 = Multiply(x=w343, y=w341) -> (x*y=w336:i32)
      n149 = String Subset(string=w351, offset (0)=2, length (rest)=1 ("length (rest)")) -> (substring=w349:string)
      n150 = Equal?(x=w389, y="Z" ("format string")) -> (x = y?=w375:bool)
      n151 = Equal?(x=w373, y=w353) -> (x = y?=w374:bool)
      n152 = String To Byte Array(string=w348) -> (unsigned byte array=w381:u8[])
      n153 = String To Byte Array(string=w347) -> (unsigned byte array=w354:u8[])
      n154 = String To Byte Array(string=w349) -> (unsigned byte array=w420:u8[])
      n155 = for {
        shift-right: [w639] -> w378
        shift-left: "" ("format string") -> [w636]
        tunnel: w420 -> [w640] mode=indexing
        n156 = Number To Hexadecimal String(2:w640) -> (0:w632:string)  [unwired: 1 in]
        n157 = String Length(string=w632) -> (length=w638:i32)
        n158 = Equal?(x=w638, y=2) -> (x = y?=w635:bool)
        n159 = Concatenate Strings("0" ("format string"), w632) -> (w634:string)
        n160 = Select(t=w632, s=w635, f=w634) -> (s? t:f=w631:string)
        n161 = Concatenate Strings(w636, w631) -> (w639:string)
      }
      n162 = for {
        shift-right: [w440] -> w379
        shift-left: "" ("format string") -> [w432]
        tunnel: w381 -> [w441] mode=indexing
        n163 = Number To Hexadecimal String(2:w441) -> (0:w434:string)  [unwired: 1 in]
        n164 = String Length(string=w434) -> (length=w439:i32)
        n165 = Concatenate Strings("0" ("format string"), w434) -> (w436:string)
        n166 = Equal?(x=w439, y=2) -> (x = y?=w437:bool)
        n167 = Select(t=w434, s=w437, f=w436) -> (s? t:f=w433:string)
        n168 = Concatenate Strings(w432, w433) -> (w440:string)
      }
      n169 = for {
        shift-right: [w430] -> w357
        shift-left: "" ("format string") -> [w422]
        tunnel: w354 -> [w431] mode=indexing
        n170 = Number To Hexadecimal String(2:w431) -> (0:w424:string)  [unwired: 1 in]
        n171 = String Length(string=w424) -> (length=w429:i32)
        n172 = Concatenate Strings("0" ("format string"), w424) -> (w426:string)
        n173 = Equal?(x=w429, y=2) -> (x = y?=w427:bool)
        n174 = Select(t=w424, s=w427, f=w426) -> (s? t:f=w423:string)
        n175 = Concatenate Strings(w422, w423) -> (w430:string)
      }
      n176 = Not(x=w367) -> (.not. x?=w366:bool)
      n177 = Compound Arithmetic op=AND(w375, w374, w366) -> (w387:bool)
      n178 = Hexadecimal String To Number(string=w378, default (0uL)=u64 0 ("default (0 U32)")) -> (number=w416:u64)  [unwired: 1 in, 1 out]
      n179 = Hexadecimal String To Number(string=w379, default (0uL)=u64 0 ("default (0 U32)")) -> (number=w346:u64)  [unwired: 1 in, 1 out]
      "channel number 2" <- w346
      n180 = Hexadecimal String To Number(string=w357, default (0uL)=u64 0 ("default (0 U32)")) -> (number=w334:u64)  [unwired: 1 in, 1 out]
      "channel number 3" <- w334
      n181 = And(x=w416, y=u64 127 ("port")) -> (x .and. y?=w338:u64)
      "channel number" <- w338
      n182 = Add(x=w336, y=w338) -> (x+y=w337:u64)
      n183 = Equal To 0?(x=w337) -> (x = 0?=w402:bool)
      n184 = Equal?(x=w337, y=u64 1) -> (x = y?=w400:bool)
      n185 = case shown="True" w387 {
        tunnel: w346 -> [_ w455]
        tunnel: w407 -> [w450 w476]
        tunnel: w415 -> [w453 w485]
        tunnel: [w453 w484] -> w417
        tunnel: [w452 w481] -> w413
        tunnel: w414 -> [w452 w480]
        tunnel: w337 -> [_ w460]
        tunnel: w409 -> [w451 w479]
        tunnel: [w451 w478] -> w410
        tunnel: [w450 w477] -> w408
        tunnel: w406 -> [w449 w475]
        tunnel: [w449 w474] -> w405
        tunnel: w402 -> [_ w473]
        tunnel: w399 -> [w448 w472]
        tunnel: [w448 w471] -> w401
        tunnel: w400 -> [_ w470]
        tunnel: w398 -> [w447 w469]
        tunnel: [w447 w468] -> w397
        tunnel: w365 -> [w446 w466]
        tunnel: [w446 w465] -> w395
        tunnel: w396 -> [_ w464]
        tunnel: w393 -> [w445 w462]
        tunnel: [w445 w461] -> w392
        tunnel: w372 -> [_ w459]
        tunnel: w371 -> [_ w458]
        tunnel: w364 -> [_ w457]
        tunnel: w334 -> [_ w456]
        tunnel: w335 -> [_ w454]
        frame False {
          (unwired) FALSE
        }
        frame True {
          n186 = Index Array(array=w475, index=w460) -> (element=w467:u32)
          n187 = Greater?(x=w467, y=w457) -> (0:w463:bool)
          n188 = And(x=w455, y=u64 1023 ("port")) -> (x .and. y?=w482:u64)
          n189 = case shown="True" w463 {
            tunnel: w485 -> [w503 w592]
            tunnel: [w502 w592] -> w484
            tunnel: w482 -> [w494 w544]
            tunnel: [w501 w576] -> w481
            tunnel: w480 -> [w501 w599]
            tunnel: w476 -> [w499 _]
            tunnel: w460 -> [w497 w574]
            tunnel: w479 -> [w500 w598]
            tunnel: [w500 w597] -> w478
            tunnel: [w499 w595] -> w477
            tunnel: w467 -> [w495 _]
            tunnel: w475 -> [w498 w594]
            tunnel: [w496 w594] -> w474
            tunnel: w473 -> [_ w587]
            tunnel: w472 -> [w493 w586]
            tunnel: [w493 w585] -> w471
            tunnel: w470 -> [_ w584]
            tunnel: w469 -> [w492 w583]
            tunnel: [w492 w582] -> w468
            tunnel: w467 -> [w490 _]
            tunnel: w457 -> [w487 _]
            tunnel: w466 -> [w489 w578]
            tunnel: [w488 w578] -> w465
            tunnel: w464 -> [_ w577]
            tunnel: w462 -> [w486 w571]
            tunnel: [w486 w570] -> w461
            tunnel: w460 -> [_ w567]
            tunnel: w459 -> [_ w565]
            tunnel: w458 -> [_ w566]
            tunnel: w456 -> [_ w560]
            tunnel: w456 -> [_ w549]
            tunnel: w455 -> [_ w541]
            tunnel: w454 -> [_ w539]
            frame False {
              n190 = Equal?(x=w490, y=w487) -> (x = y?=w491:bool)
              n191 = case shown="True" w491 {
                tunnel: w503 -> [w514 w520]
                tunnel: [w512 w520] -> w502
                tunnel: w498 -> [w510 w518]
                tunnel: w497 -> [w509 w515]
                tunnel: [w507 w517] -> w496
                tunnel: w495 -> [w506 w516]
                tunnel: w494 -> [w505 _]
                tunnel: w489 -> [w504 w522]
                tunnel: [w504 w521] -> w488
                frame False {
                  n192 = Index Array(array=w514, index (row)=w505, index (col)=w509) -> (element=w513:u32)
                  n193 = Increment(x=w513) -> (x+1=w511:u32)
                  n194 = Replace Array Subset(array=w514, new element=w511, index (row)=w505, index (col)=w509) -> (w512:u32[][])
                  n195 = Increment(x=w506) -> (x+1=w508:u32)
                  n196 = Replace Array Subset(array=w510, new element=w508, index=w509) -> (w507:u32[])
                  "Calibration Counter" <- w506
                }
                frame True {
                  n197 = for {
                    N: 2048 -> [_]
                    tunnel: w520 -> [w532]
                    tunnel: w515 -> [w525]
                    shift-right: [w527] -> w521
                    shift-left: w522 -> [w528]
                    i -> [w524]
                    n198 = Array Subset(array=w532, index (row)=0 ("索引"), length (row)=w524, index (col)=w525, length (col)=1 ("长度")) -> (w529:u32[][])
                    n199 = Add Array Elements(numeric array=w529) -> (sum=w526:u32)
                    n200 = Replace Array Subset(array=w528, new element=w526, index (row)=w524, index (col)=w525) -> (w527:u32[][])
                  }
                  n201 = Increment(x=w516) -> (x+1=w519:u32)
                  n202 = Replace Array Subset(array=w518, new element=w519, index=w515) -> (w517:u32[])
                }
              }
            }
            frame True {
              (unwired) 0.0 ("x")
              w589 = 0 ("索引 (行)")
              w591 = 1 ("长度")
              # "正式取数"
              n203 = And(x=w549, y=u64 31 ("port")) -> (x .and. y?=w557:u64)
              n204 = And(x=w560, y=u64 63 ("port")) -> (x .and. y?=w563:u64)
              n205 = Logical Shift(y=i16 -13, x=w563) -> (x << y=w545:u64)
              n206 = Logical Shift(y=i16 -19, x=w557) -> (x << y=w556:u64)
              n207 = And(x=w549, y=u64 63 ("port")) -> (x .and. y?=w537:u64)
              n208 = And(x=w541, y=w539) -> (x .and. y?=w540:u64)
              "fine 4" <- w540
              n209 = Multiply(x=u64 3600, y=w556) -> (x*y=w552:u64)
              n210 = Logical Shift(y=i16 -8, x=w540) -> (x << y=→"fine 3":u64)
              n211 = Multiply(x=u64 60, y=w545) -> (x*y=w553:u64)
              n212 = Logical Shift(y=i16 -10, x=w540) -> (x << y=w534:u64)
              "fine 2" <- w534
              n213 = Add(x=w553, y=w552) -> (x+y=w551:u64)
              n214 = Logical Shift(y=i16 -7, x=w537) -> (x << y=w536:u64)
              n215 = Add(x=w551, y=w536) -> (x+y=w535:u64)
              "x+y" <- w535
              n216 = Add(x=w534, y=w535) -> (x+y=w533:u64)
              n217 = Equal?(x=w567, y=u32 2) -> (x = y?=w569:bool)
              n218 = case shown="True" w569 {
                tunnel: w571 -> [w604 w607]
                tunnel: w533 -> [_ w606]
                tunnel: [w604 w605] -> w570
                frame False {
                }
                frame True {
                  n219 = Build Array (concatenate)(w607, w606) -> (w605:u64[])
                }
              }
              "cal 2" <- w570
              n220 = case shown="True" TRUE {
                tunnel: [w614 w622] -> w601
                tunnel: w592 -> [_ _]
                tunnel: w574 -> [w619 w620]
                tunnel: w544 -> [w617 w625]
                tunnel: w578 -> [w618 w626]
                frame False {
                  w613 = 0 ("index (row)")
                  w616 = 1 ("长度")
                  n221 = Decrement(x=w619) -> (x-1=w612:u64)
                  n222 = Array Subset(array=w618, index (row)=w617, length (row)=w616, index (col)=w612, length (col)=w616) -> (w615:u32[][])
                  n223 = Index Array(array=w615, index (row)=w613, index (col)=w613) -> (element=w614:u32)
                }
                frame True {
                  w621 = 0 ("index (row)")
                  w624 = 1 ("长度")
                  n224 = Array Subset(array=w626, index (row)=w625, length (row)=w624, index (col)=w620, length (col)=w624) -> (w623:u32[][])
                  n225 = Index Array(array=w623, index (row)=w621, index (col)=w621) -> (element=w622:u32)
                }
              }
              n226 = Multiply(x=w533, y=w565) -> (x*y=w548:dbl)
              n227 = Index Array(array=w598, index=w574) -> (element=w595:u32)
              n228 = Array Subset(array=w592, index (row)=w544, length (row)=w591, index (col)=w574, length (col)=w591) -> (w590:u32[][])
              n229 = Index Array(array=w590, index (row)=w589, index (col)=w589) -> (element=w588:u32)
              n230 = Divide(x=w588, y=u32 2) -> (x/y=w593:dbl)
              n231 = Increment(x=w595) -> (x+1=w596:u32)
              n232 = Add(x=w601, y=w593) -> (x+y=w600:dbl)
              n233 = Add(x=w548, y=0.0) -> (x+y=w547:dbl)
              n234 = Multiply(x=w600, y=w566) -> (x*y=w580:dbl)
              n235 = Subtract(x=w565, y=w580) -> (x-y=w564:dbl)
              n236 = Add(x=w564, y=w547) -> (x+y=w581:dbl)
              n237 = Replace Array Subset(array=w598, new element=w596, index=w574) -> (w597:u32[])
              n238 = case shown="True" w587 {
                tunnel: w581 -> [_ w630]
                tunnel: [w629 w630] -> w585
                tunnel: w586 -> [w629 _]
                frame False {
                }
                frame True {
                }
              }
              n239 = case shown="False" w584 {
                tunnel: [w627 w628] -> w582
                tunnel: w583 -> [w627 _]
                tunnel: w581 -> [_ w628]
                frame False {
                }
                frame True {
                }
              }
              n240 = Replace Array Subset(array=w599, new element=w581, index=w574) -> (w575:dbl[])
              n241 = case shown="True" "save data" {
                tunnel: w577 -> [_ w611]
                tunnel: w575 -> [_ w609]
                frame False {
                }
                frame True {
                  n242 = call-poly <vilib>:"Write Delimited Spreadsheet.vi"("file path (dialog if empty)"=w611, "1D data"=w609, "append to file? (new file:F)"="append csv", "delimiter (\\t)"="," ("delimiter (\\t)")) -> ()  [unwired: 10 in, 2 out]
                }
              }
              n243 = Replace Array Subset(array=w575, new element=0.0 ("new element/subarray"), index=w574) -> (w576:dbl[])
              "fine" <- w544
            }
          }
        }
      }
    }
    n244 = case shown="True" "RST" {
      tunnel: w230 -> [w331 _]
      tunnel: [w331 0] -> w253
      tunnel: [w330 w332] -> w251
      tunnel: w231 -> [w330 _]
      frame False {
      }
      frame True {
        n245 = Get Date/Time In Seconds() -> (seconds since 1Jan1904=w332:timestamp)
      }
    }
  }
  "error out 2" <- w53
  n246 = Close File(refnum=w43, error in=w79) -> (error out=→"error out":errorcluster)  [unwired: 1 out]
  n247 = call-poly <vilib>:"Write Delimited Spreadsheet.vi"("file path (dialog if empty)"=w56, "2D data"=w57, "append to file? (new file:F)"=FALSE, "transpose? (no:F)"=TRUE, "delimiter (\\t)"="," ("delimiter (\\t)")) -> ()  [unwired: 9 in, 2 out]
